vi "JKISM Module Async-Call.vi"() -> ()   [LabVIEW 2014]
uses:
  user.lib/_NEVSTOP/JKI State Machine++/_Support/JKISMQ/_Create Data Queue.vi
  user.lib/_NEVSTOP/JKI State Machine++/JKI State Machine++.lvlib
panel:
  out "error":errorcluster
  in  "Stop Module":bool
  in  "Start Module":bool
  out "Exist?":bool
  in  "DoSth: DoC(error)":bool
  in  "DoSth: DoB":bool
  in  "DoSth: DoA":bool
  # "Start/Stop Module"
  # "Module Message"
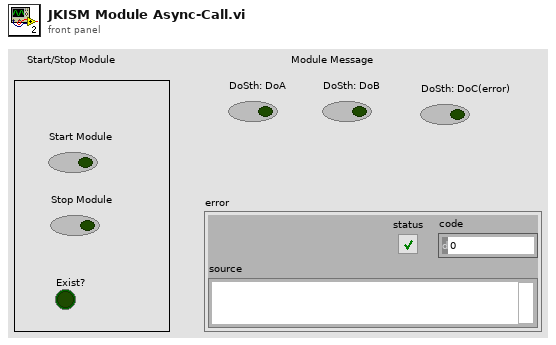
[diagram p1: front panel]
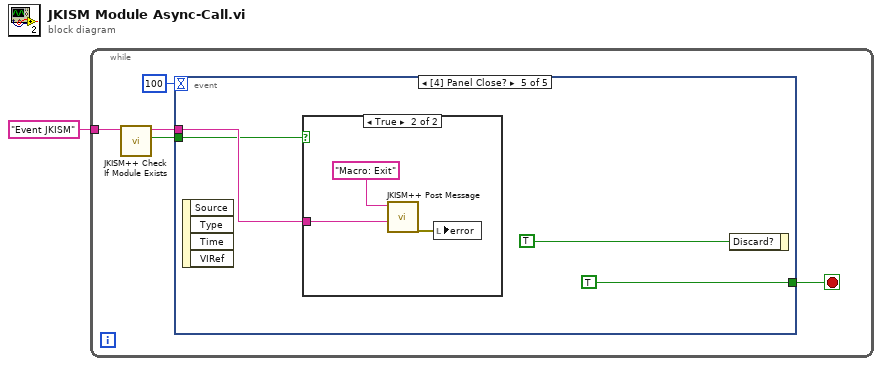
[diagram p0: block diagram]
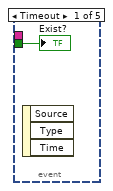
[diagram p2: hidden frame]
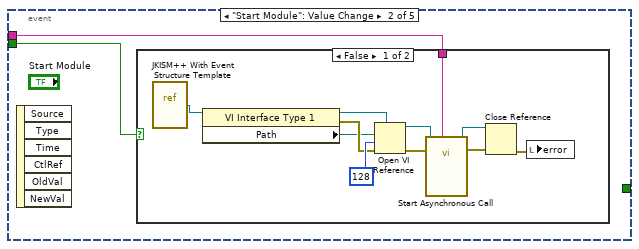
[diagram p3: hidden frame]
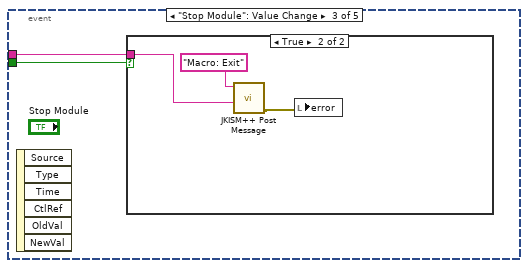
[diagram p5: hidden frame]
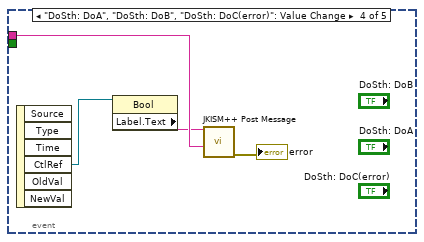
[diagram p7: hidden frame]
diagram:
  n1 = while {
    tunnel: "Event JKISM" ("Name(\"\" to use uuid)") -> [w4]
    stop <- w6 stop-if-true
    n2 = call "JKISM++ Check If Module Exists.vi"("JKISM Name"=w4) -> ("Exist?"=w2:bool, "JKISM Name(dup)"=w3:string)  [unwired: 8 in, 1 out]
    n3 = event shown="[4] Panel Close?" {
      selector: _ -> [_ _ _ _ _]
      dyn-events: _ -> [_ _ _ _ _]
      timeout: 100 -> [_ _ _ _ _]
      tunnel: [_ _ _ _ TRUE ("Discard?")] -> w6
      tunnel: w3 -> [_ w8 w21 w29 w31]
      tunnel: w2 -> [w7 w9 w22 _ w30]
      event Timeout {
        n4 = event-data() -> ()  [unwired: 1 in, 3 out]
        "Exist?" <- w7
      }
      event "Start Module": Value Change {
        n5 = event-data() -> ()  [unwired: 1 in, 6 out]
        n6 = case shown="False" w9 {
          tunnel: w8 -> [w11 _]
          frame False {
            n7 = vi-ref "JKISM++ With Event Structure Template.vi"() -> (w13:refnum<vi>)
            n8 = property class="VI Interface Type 1"(reference=w13) -> (reference out=w17:refnum<vi>, error out=w15:errorcluster, "Path"=w14:path)  [unwired: 1 in]
            n9 = Open VI Reference(type specifier VI Refnum (for type only)=w17, vi path=w14, options=128, error in (no error)=w15) -> (vi reference=w16:refnum<vi>, error out=w12:errorcluster)  [unwired: 2 in]
            n10 = call-by-ref "Start Asynchronous Call"(reference=w16, error in=w12, "Name(\"\" to use uuid)"=w11) -> (reference out=w19:refnum<vi>, error out=w18:errorcluster)  [unwired: 11 in]
            n11 = Close Reference(reference=w19, error in (no error)=w18) -> (error out=w10:errorcluster)
            n12 = local write "error"(w10) -> ()
          }
          frame True {
          }
        }
      }
      event "Stop Module": Value Change {
        n13 = event-data() -> ()  [unwired: 1 in, 6 out]
        n14 = case shown="True" w22 {
          tunnel: w21 -> [_ w25]
          frame False {
          }
          frame True {
            n15 = call "JKISM++ Post Message.vi"("Target Module"=w25, "State"="Macro: Exit" ("States")) -> ("error out"=w23:errorcluster)  [unwired: 9 in]
            n16 = local write "error"(w23) -> ()
          }
        }
      }
      event "DoSth: DoA", "DoSth: DoB", "DoSth: DoC(error)": Value Change {
        n17 = event-data() -> ("CtlRef"=w28:refnum<vi>)  [unwired: 1 in, 5 out]
        n18 = property class="Bool"(reference=w28) -> ("Label.Text"=w27:string)  [unwired: 1 in, 2 out]
        n19 = call "JKISM++ Post Message.vi"("Target Module"=w29, "State"=w27) -> ("error out"=→"error":errorcluster)  [unwired: 9 in]
      }
      event Panel Close? {
        n20 = event-data() -> ()  [unwired: 1 in, 4 out]
        n21 = case shown="True" w30 {
          tunnel: w31 -> [_ w35]
          frame False {
          }
          frame True {
            n22 = call "JKISM++ Post Message.vi"("Target Module"=w35, "State"="Macro: Exit" ("States")) -> ("error out"=w34:errorcluster)  [unwired: 9 in]
            n23 = local write "error"(w34) -> ()
          }
        }
        n24 = event-data("Discard?"=TRUE) -> ()  [unwired: 1 in, 1 out]
      }
    }
  }
